vi "test child test method.vi"(8 "error in (no error)":errorcluster, 11 "LUnit child class in":refnum<class "LUnit child class.lvclass">) -> (0 "error out":errorcluster, 3 "LUnit child class out":refnum<class "LUnit child class.lvclass">)   [LabVIEW 2020, in "LUnit child class.lvclass"]
uses:
  LUnit child class.lvclass
  C:/Program Files (x86)/National Instruments/LabVIEW 2020/vi.lib/Astemes/LUnit/Test Case.lvclass
  <vilib>/Astemes/LUnit/Test Case.lvclass/Test Case.ctl
  <vilib>/Astemes/LUnit/Append Fail Result.vi
  <vilib>/Astemes/LUnit/Append Pass Result.vi
  <vilib>/Astemes/LUnit/Run In UI.vi
  <vilib>/Utility/error.llb/Clear Errors.vi
  <vilib>/Astemes/LUnit/Test Case.lvclass
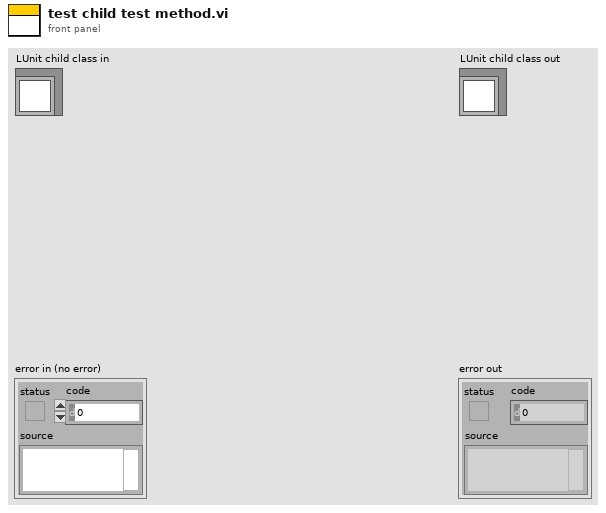
[diagram p1: front panel]
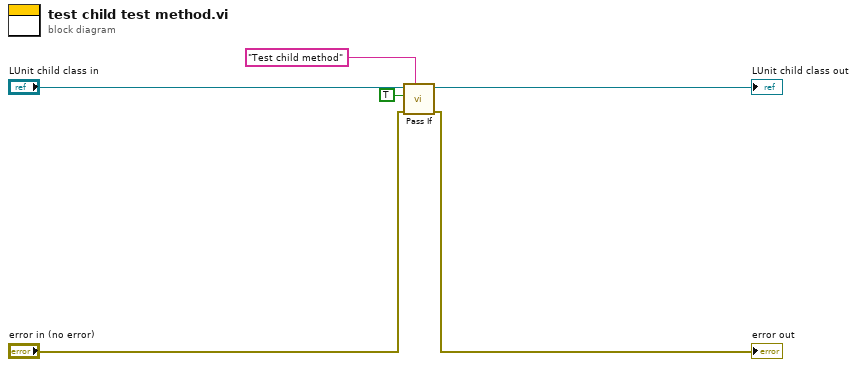
[diagram p0: block diagram]
diagram:
  n1 = call <vilib>:"Pass If.vi"("Description"="Test child method", "error in (no error)"="error in (no error)", "Pass?"=TRUE, "LUnit Test Case In"="LUnit child class in") -> ("error out"=→"error out":errorcluster, "LUnit Test Case Out"=→"LUnit child class out":refnum<class "LUnit child class.lvclass">)  [unwired: 6 in]
